vi "simple_read.vi"() -> ()   [LabVIEW 2024]
uses:
  <vilib>/Instr/_visa.llb/VISA Configure Serial Port (Instr).vi
panel:
  in  "Stop":bool
  in  "VISA resource name 2":refnum<visa-resource-name>
  out "Array - String":string[](array[string])
  out "String":string
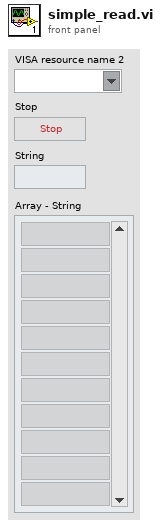
[diagram p1: front panel]
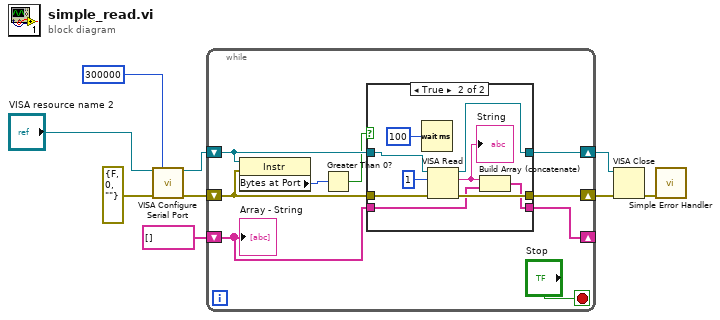
[diagram p0: block diagram]
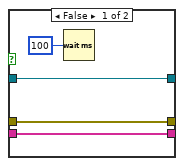
[diagram p2: hidden frame]
diagram:
  n1 = call-poly "VISA Configure Serial Port"("VISA resource name"="VISA resource name 2", "timeout (10sec)"=u32 300000, "error in (no error)"=errorcluster {"status"=FALSE, "code"=0, "source"=""}) -> ("VISA resource name out"=w9:refnum<visa-resource-name>, "error out"=w8:errorcluster)  [unwired: 11 in]
  n2 = while {
    shift-right: [w10] -> _
    shift-left: string[] [] -> [w11]
    shift-right: [w18] -> w5
    shift-left: w9 -> [w16]
    shift-right: [w17] -> w6
    shift-left: w8 -> [w15]
    stop <- "Stop" stop-if-true
    n3 = property class="Instr"(reference=w16, error in=w15) -> ("Bytes at Port"=w14:u32)  [unwired: 2 out]
    n4 = Greater Than 0?(x=w14) -> (x > 0?=w13:bool)
    n5 = case shown="True" w13 {
      tunnel: [w21 w31] -> w18
      tunnel: [w20 w30] -> w17
      tunnel: w16 -> [w21 w27]
      tunnel: w15 -> [w20 w26]
      tunnel: w11 -> [w19 w24]
      tunnel: [w19 w23] -> w10
      frame False {
        n6 = Wait (ms)(milliseconds to wait=u32 100) -> ()  [unwired: 1 out]
      }
      frame True {
        n7 = Wait (ms)(milliseconds to wait=u32 100) -> ()  [unwired: 1 out]
        n8 = VISA Read(VISA resource name=w27, byte count=u32 1, error in (no error)=w26) -> (VISA resource name out=w31:refnum<visa-resource-name>, read buffer=w28:string, error out=w30:errorcluster)  [unwired: 1 out]
        "String" <- w28
        n9 = Build Array (concatenate)(w28, w24) -> (w23:string[])
      }
    }
    "Array - String" <- w11
  }
  n10 = VISA Close(VISA resource name=w5, error in (no error)=w6) -> (error out=w3:errorcluster)
  n11 = call <vilib>:"Simple Error Handler.vi"("error in (no error)"=w3) -> ()  [unwired: 4 in, 5 out]
